vi "testing.vi"() -> ()   [LabVIEW 2021]
uses:
  Lab 3 Template/State.ctl
  <vilib>/Math Plots/2D Math Plots/2D Compass/2D Compass Datatype/2D Compass Datatype.lvclass
  <vilib>/Math Plots/2D Math Plots/2D Plot/2D Plot Datatype/2D Plot Datatype.lvclass
  <vilib>/Math Plots/2D Math Plots/2D Compass/2D Compass Datatype/Public/Plot Helper (Vector).vi
  <vilib>/Math Plots/2D Math Plots/2D Compass/2D Compass XCtrl/2D Compass.xctl
panel:
  out "2D Compass":refnum<class "2D Plot Datatype.lvclass">[](xcontrol)
  out "Intensity Chart":dbl[][](graph)
  out "Thermometer":dbl(slide) scale=0.0..100.0
  in  "stop":bool
  # "https://www.youtube.com/watch?v=bWew4fHWVKo"
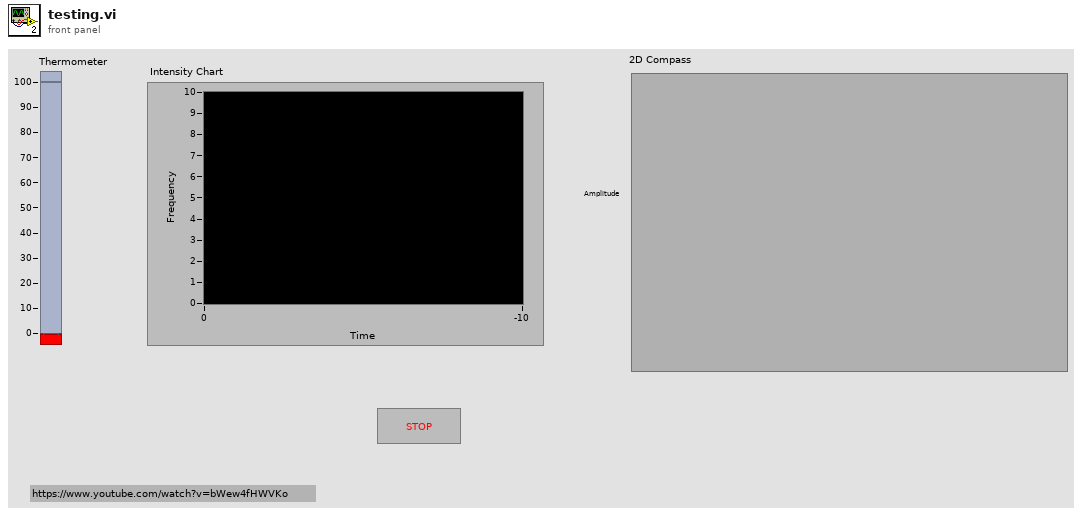
[diagram p1: front panel]
types:
  T1 = typedef "State.ctl" = enum16{"Reset", "Initialize", "Wait", "Shutdown"}
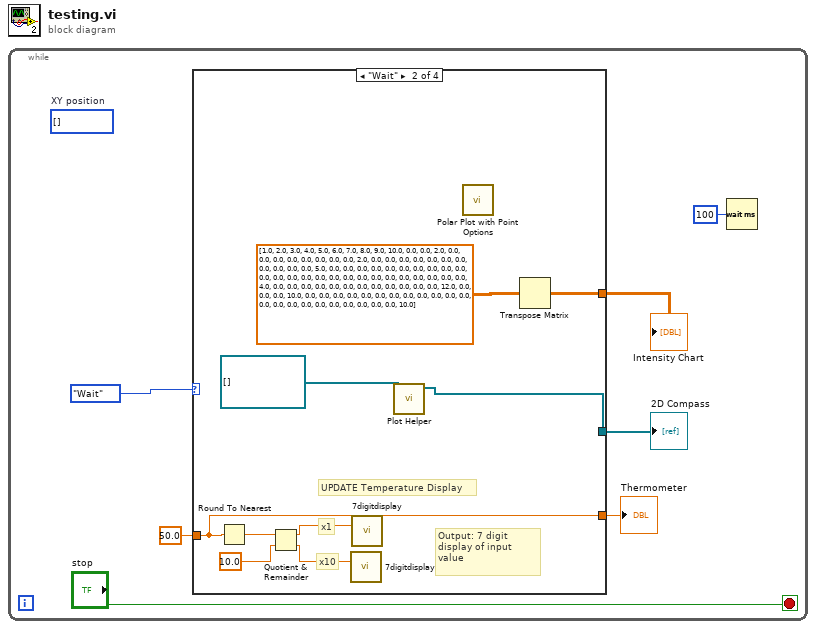
[diagram p0: block diagram]
diagram:
  n1 = while {
    stop <- "stop" stop-if-true
    (unwired) i32[] []  # XY position
    n2 = case shown="\"Wait\"" State."Wait" {
      tunnel: 50.0 ("Thermometer") -> [_ w12 _ _]
      tunnel: [_ w12 _ _] -> w4
      tunnel: [_ w11 _ _] -> w2
      tunnel: [_ w9 _ _] -> w1
      frame "Initialize", Default {
      }
      frame "Wait" {
        # "Output: 7 digit display of input value"
        # "UPDATE Temperature Display"
        # "x10"
        # "x1"
        n3 = Round To Nearest(number=w12) -> (nearest integer value=w15:dbl)
        n4 = Quotient & Remainder(x=w15, y=10.0) -> (x-y*floor(x/y)=w14:dbl, floor(x/y)=w13:dbl)
        n5 = call "7digitdisplay.vi"("Numeric"=w13) -> ()  [unwired: 14 in, 1 out]
        n6 = call "7digitdisplay.vi"("Numeric"=w14) -> ()  [unwired: 14 in, 1 out]
        n7 = call-poly <vilib>:"Plot Helper.vi"("2D Plot Class Obj Array in"=refnum<class "2D Plot Datatype.lvclass">[] []) -> ("2D Plot Class Obj Array out"=w9:refnum<class "2D Plot Datatype.lvclass">[])  [unwired: 3 in, 7 out]
        n8 = call <vilib>:"Polar Plot with Point Options.vi"() -> ()  [unwired: 15 in, 1 out]
        n9 = Transpose Matrix(1:dbl[][] [[1.0, 2.0, 3.0, 4.0, 5.0, 6.0, 7.0, 8.0, 9.0, 10.0], [0.0, 0.0, 2.0, 0.0, 0.0, 0.0, 0.0, 0.0, 0.0, 0.0], [0.0, 2.0, 0.0, 0.0, 0.0, 0.0, 0.0, 0.0, 0.0, 0.0], [0.0, 0.0, 0.0, 5.0, 0.0, 0.0, 0.0, 0.0, 0.0, 0.0], [0.0, 0.0, 0.0, 0.0, 0.0, 0.0, 0.0, 0.0, 0.0, 0.0], [0.0, 0.0, 0.0, 0.0, 0.0, 0.0, 0.0, 0.0, 0.0, 4.0], [0.0, 0.0, 0.0, 0.0, 0.0, 0.0, 0.0, 0.0, 0.0, 0.0], [0.0, 0.0, 12.0, 0.0, 0.0, 0.0, 10.0, 0.0, 0.0, 0.0], [0.0, 0.0, 0.0, 0.0, 0.0, 0.0, 0.0, 0.0, 0.0, 0.0], [0.0, 0.0, 0.0, 0.0, 0.0, 0.0, 0.0, 0.0, 0.0, 10.0]] ("Intensity Chart")) -> (0:w11:dbl[][])
      }
      frame "Shutdown" {
      }
      frame "Reset" {
      }
    }
    "Intensity Chart" <- w2
    "Thermometer" <- w4
    "2D Compass" <- w1
    n10 = Wait (ms)(milliseconds to wait=u32 100) -> ()  [unwired: 1 out]
  }
